vi "Return Home.vi"(6 "chip select (1st chip)":enum16{"1st chip", "2nd chip"}(ring), 8 "error in (no error)":errorcluster, 11 "LCD in":u32) -> (0 "error out":errorcluster, 3 "LCD out":u32)   [LabVIEW 2015, in "HD44780 FPGA.lvlib"]
doc: "Returns the cursor to the home position and shift the display to the original position. This VI sets the current address to display data RAM (DDRAM) 0. The DDRAM contents remain unchanged."
uses:
  <vilib>/EmbeddedDisplay/Hitachi HD44780/FPGA/HD44780 FPGA.lvlib
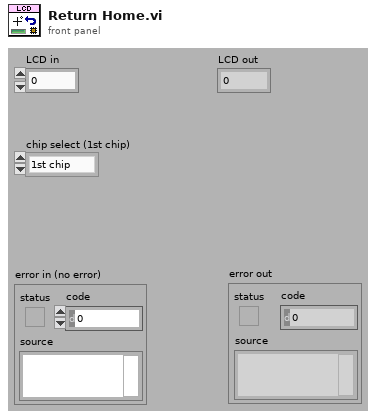
[diagram p1: front panel]
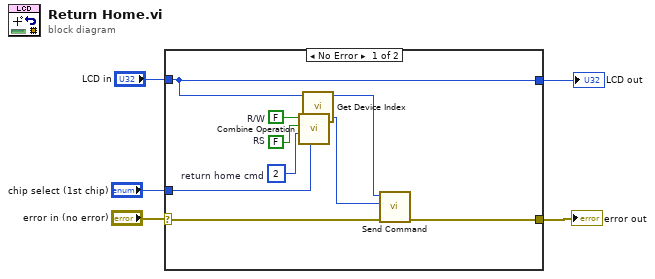
[diagram p0: block diagram]
diagram:
  n1 = case shown="No Error" "error in (no error)" {
    selector: "error in (no error)" -> [w10 w16]
    tunnel: [w8 w16] -> w4
    tunnel: "LCD in" -> [w6 w15]
    tunnel: [w6 w15] -> w2
    tunnel: "chip select (1st chip)" -> [w9 _]
    frame No Error {
      w12 = FALSE  # R/W
      w14 = u8 2  # return home cmd
      w13 = FALSE  # RS
      n2 = call <vilib>:"Combine Operation.vi"("chip select  (1st chip)"=w9, "cmd/data (0)"=w14, "RS"=w13, "R/W"=w12) -> ("output"=w11:u32)  [unwired: 7 in]
      n3 = call <vilib>:"Get Device Index.vi"("LCD in"=w6) -> ("device index"=w7:i8)  [unwired: 10 in]
      n4 = call <vilib>:"Send Command.vi"("error in (no error)"=w10, "operation"=w11, "device index"=w7) -> ("error out"=w8:errorcluster)  [unwired: 6 in, 2 out]
    }
    frame Error {
    }
  }
  "error out" <- w4
  "LCD out" <- w2
